vi "AB_1200_1100_Project_DLL_Info.vi"(7 "action":T1, 8 "error in (no error)":errorcluster, 10 "Dll_info in":T2, 11 "Object In":T3) -> (0 "error out":errorcluster, 2 "Dll info out":T2, 3 "Object Out":T3)   [LabVIEW 2020]
uses:
  <resource>/Framework/Providers/API/ItemRef.ctl
  <vilib>/AppBuilder/RW_Project/AB_RW_Project_PropBag_Action.ctl
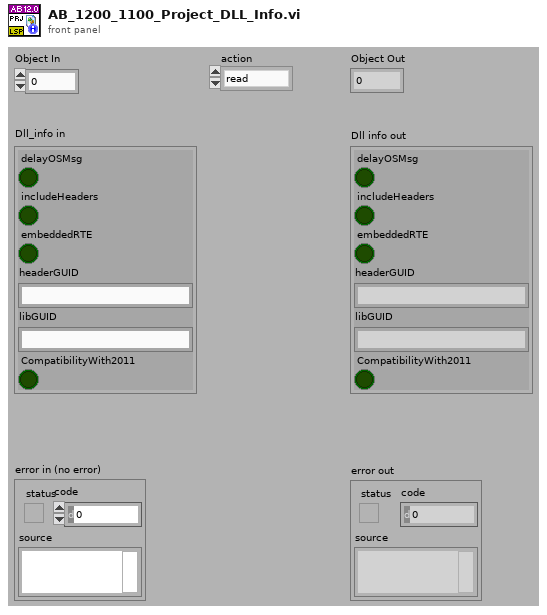
[diagram p1: front panel]
types:
  T1 = typedef "AB_RW_Project_PropBag_Action.ctl" = enum16{"read", "write", "clear", "readPrevious", "writePrevious", "clearPrevious"}
  T2 = cluster{"delayOSMsg":bool, "includeHeaders":bool, "embeddedRTE":bool, "headerGUID":string, "libGUID":string, "CompatibilityWith2011":bool}
  T3 = typedef "ItemRef.ctl" = u64
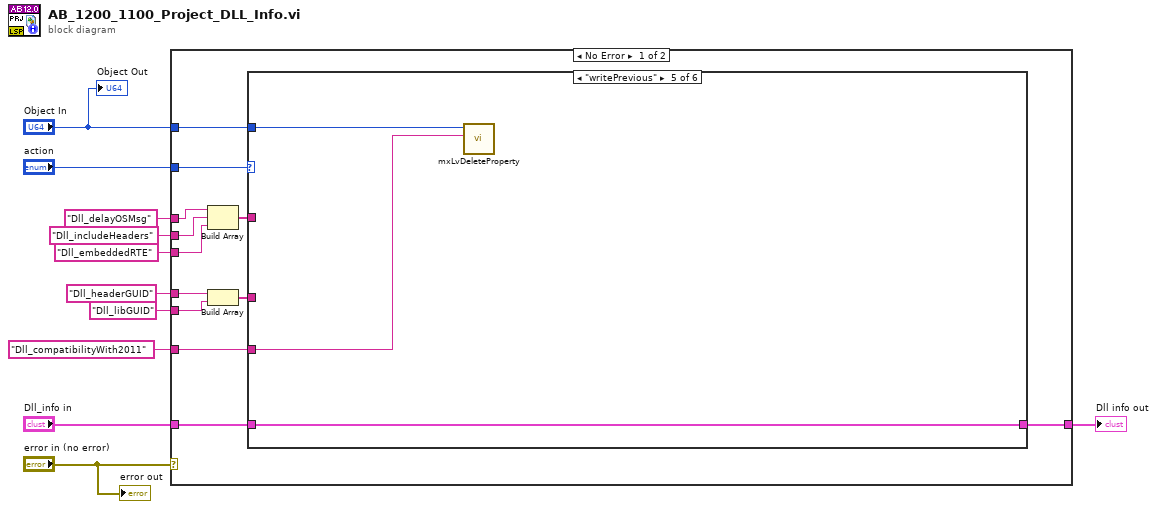
[diagram p0: block diagram]
diagram:
  n1 = case shown="No Error" "error in (no error)" {
    tunnel: "Object In" -> [w22 _]
    tunnel: [w23 _] -> w9
    tunnel: "Dll_info in" -> [w21 _]
    tunnel: "action" -> [w20 _]
    tunnel: "Dll_delayOSMsg" -> [w19 _]
    tunnel: "Dll_includeHeaders" ("Tag") -> [w18 _]
    tunnel: "Dll_embeddedRTE" ("Tag") -> [w17 _]
    tunnel: "Dll_headerGUID" -> [w16 _]
    tunnel: "Dll_libGUID" -> [w15 _]
    tunnel: "Dll_compatibilityWith2011" -> [w12 _]
    frame No Error {
      n2 = Build Array(w19, w18, w17) -> (w14:string[])
      n3 = Build Array(w16, w15) -> (w13:string[])
      n4 = case shown="\"writePrevious\"" w20 {
        tunnel: [w24 w25 w26 w27 w30 w31] -> w23
        tunnel: w22 -> [_ _ _ _ w28 _]
        tunnel: w21 -> [w24 w25 w26 w27 w30 w31]
        tunnel: w14 -> [_ _ _ _ _ _]
        tunnel: w13 -> [_ _ _ _ _ _]
        tunnel: w12 -> [_ _ _ _ w29 _]
        frame "read" {
        }
        frame "write" {
        }
        frame "clear" {
        }
        frame "readPrevious" {
        }
        frame "writePrevious" {
          n5 = call <resource>:"mxLvDeleteProperty.vi"("Tag"=w29, "Item"=w28) -> ()  [unwired: 8 in, 2 out]
        }
        frame "clearPrevious" {
        }
      }
    }
    frame Error {
    }
  }
  "Dll info out" <- w9
  "Object Out" <- "Object In"
  "error out" <- "error in (no error)"
